vi "CSInterface.vi"() -> ()   [LabVIEW 2010]
uses:
  C:/Users/xkenneth/Work/lvcstut1/CSInterface/LabVIEWInterface.dll
  LabVIEWInterface.dll
panel:
  in  "x":dbl
  out "MyCos":dbl
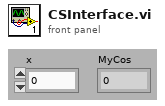
[diagram p1: front panel]
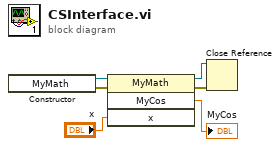
[diagram p0: block diagram]
diagram:
  n1 = constructor class="MyMath"() -> (reference out=w6:refnum<k24>, error out=w5:errorcluster)  [unwired: 3 in, 1 out]
  n2 = invoke class="MyMath" method="MyCos"(reference=w6, error in=w5, "x"="x") -> (reference out=w1:refnum<k24>, error out=w2:errorcluster, "MyCos"=→"MyCos":dbl)  [unwired: 1 in, 1 out]
  n3 = Close Reference(reference=w1, error in (no error)=w2) -> ()  [unwired: 1 out]
